vi "FitCurveSimple.vi"() -> ()   [LabVIEW 2016]
uses:
  <vilib>/Analysis/1siggen.llb/Ramp Pattern by Samples.vi
  <vilib>/gmath/NumericalOptimization/Nonlinear Curve Fit LM.vi
  <vilib>/gmath/NI_Gmath.lvlib
  <vilib>/Analysis/NI_AALBase.lvlib
panel:
  out "Best Fit parameters":dbl[](array[numeric]) caption="Offset\n\nAmplitude\n\nTime constant"
  in  "Parameter Guess":dbl[](array[numeric])=[0.0, 2.0, 0.5] caption="Offset\n\nAmplitude\n\nTime constant"
  in  "Noise":dbl=0.02
  in  "Simulation parameters":dbl[](array[numeric])=[0.2, 3.0, 0.3] caption="Offset\n\nAmplitude\n\nTime constant"
  out "error out":errorcluster
  in  "stop":bool
  out "XY Graph":cluster{cdb[]}[](graph)
  # "This demo simulates noisy data\nReplace with your experimental data!"
  # "- Run VI\n- Change simulation parameters\n- Change Noise\n- Change Guess\n\n- Watch the quality of the fit."
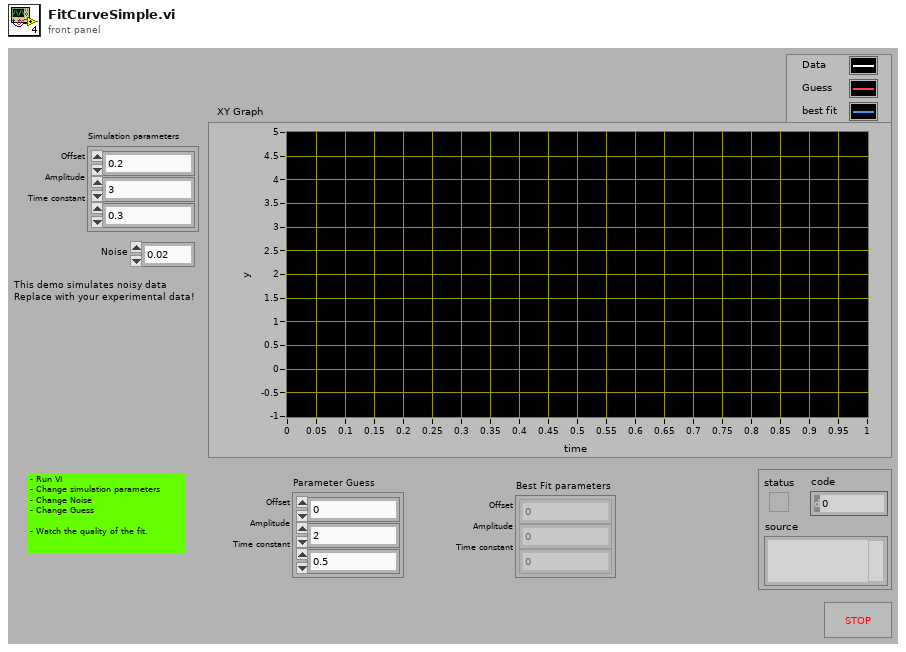
[diagram p1: front panel]
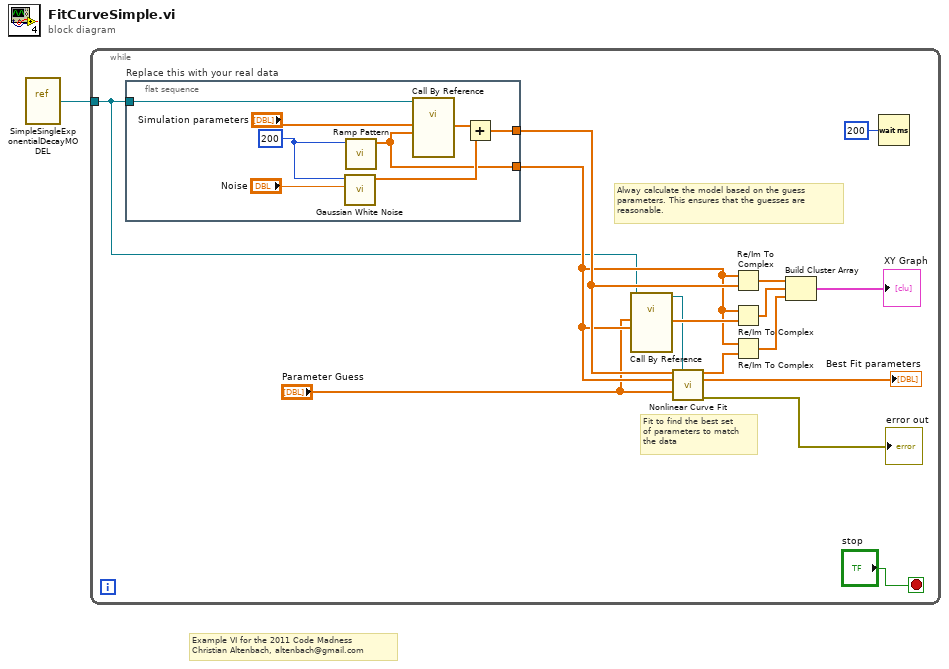
[diagram p0: block diagram]
diagram:
  # "Example VI for the 2011 Code Madness\nChristian Altenbach, altenbach@gmail.com"
  n1 = vi-ref "SimpleSingleExponentialDecayMODEL.vi"() -> (w1:refnum<vi>)
  n2 = while {
    tunnel: w1 -> [w4]
    stop <- "stop" stop-if-true
    # "Fit to find the best set\nof parameters to match\nthe data"
    # "Alway calculate the model based on the guess\nparameters. This ensures that the guesses are\nreasonable."
    n3 = flat-sequence "Replace this with your real data" {
      tunnel: [w20] -> w6
      tunnel: [w18] -> w5
      tunnel: w4 -> [w17]
      frame #0 {
        w24 = 200 ("samples")
        n4 = call <vilib>:"Gaussian White Noise.vi"("standard deviation"="Noise", "samples"=w24) -> ("Gaussian noise pattern"=w22:dbl[])  [unwired: 8 in, 1 out]
        n5 = call-poly <vilib>:"Ramp Pattern.vi"("samples"=w24) -> ("Ramp Pattern"=w18:dbl[])  [unwired: 9 in, 1 out]
        n6 = call-by-ref "?"(reference=w17, "frequency"=w18, "tau"="Simulation parameters") -> ("Phase"=w23:dbl[])  [unwired: 3 in, 4 out]
        n7 = Add(x=w23, y=w22) -> (x+y=w20:dbl[])
      }
    }
    n8 = call-by-ref "?"(reference=w4, "frequency"=w5, "tau"="Parameter Guess") -> (reference out=w9:refnum<vi>, "Phase"=w11:dbl[])  [unwired: 3 in, 3 out]
    n9 = call-poly <vilib>:"Nonlinear Curve Fit.vi"("Y"=w6, "f(x,a)"=w9, "X"=w5, "initial parameters"="Parameter Guess") -> ("best nonlinear fit"=w14:dbl[], "best fit parameters"=→"Best Fit parameters":dbl[], "error out"=→"error out":errorcluster)  [unwired: 6 in, 3 out]
    n10 = Re/Im To Complex(1:w6, 2:w5) -> (0:w16:cdb[])
    n11 = Re/Im To Complex(1:w11, 2:w5) -> (0:w13:cdb[])
    n12 = Re/Im To Complex(1:w14, 2:w5) -> (0:w12:cdb[])
    n13 = Build Cluster Array(w16, w13, w12) -> (→"XY Graph":cluster{cdb[]}[])
    n14 = Wait (ms)(milliseconds to wait=u32 200) -> ()  [unwired: 1 out]
  }
